vi "Buffer Statistics.vi"(0 "VISA resource name":refnum<visa-resource-name>, 5 "Channel (Channel A)":enum8{"Channel A", "Channel B"}(ring), 7 "Reading Buffer":string, 11 "error in (no error)":errorcluster) -> (4 "VISA resource name out":refnum<visa-resource-name>, 6 "Minimum Reading Details":string[](array[string]), 8 "Maximum Reading Details":string[](array[string]), 15 "error out":errorcluster)   [LabVIEW 2018, in "Keithley 2600 Series.lvlib"]
doc: "This Vi will return a table with statistical data about the data inserted into the buffer. \n\n<b>Functions and Attributes used</b>\nsmux.buffer.recalculatestats\nsmux.buffer.getstats"
uses:
  Keithley 2600 Series.lvlib
  Private/GlobalVariables.vi
panel:
  out "Statistics Undefined":bool
  out "Standard Deviation":dbl
  out "Mean":dbl
  out "Number of Data Points":u32
  # "(c) 2010 Keithley Instruments, Inc.  ALL RIGHTS RESERVED."
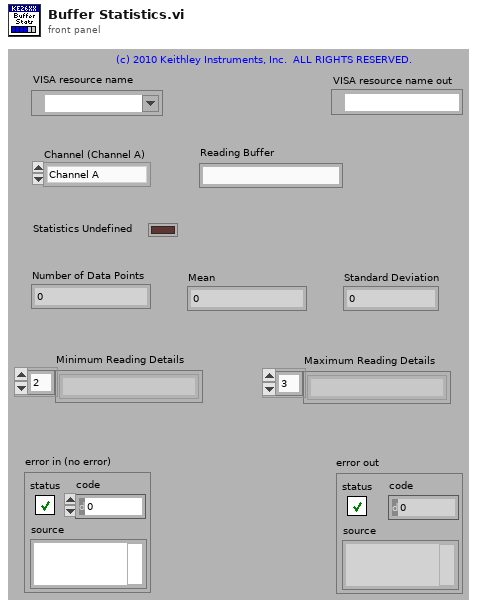
[diagram p1: front panel]
types:
  T1 = cluster{"[0]":dbl, "[1]":dbl, "[2]":dbl, "[3]":dbl, "[4]":dbl, "[5]":dbl, "[6]":dbl, "[7]":dbl, "[8]":dbl}
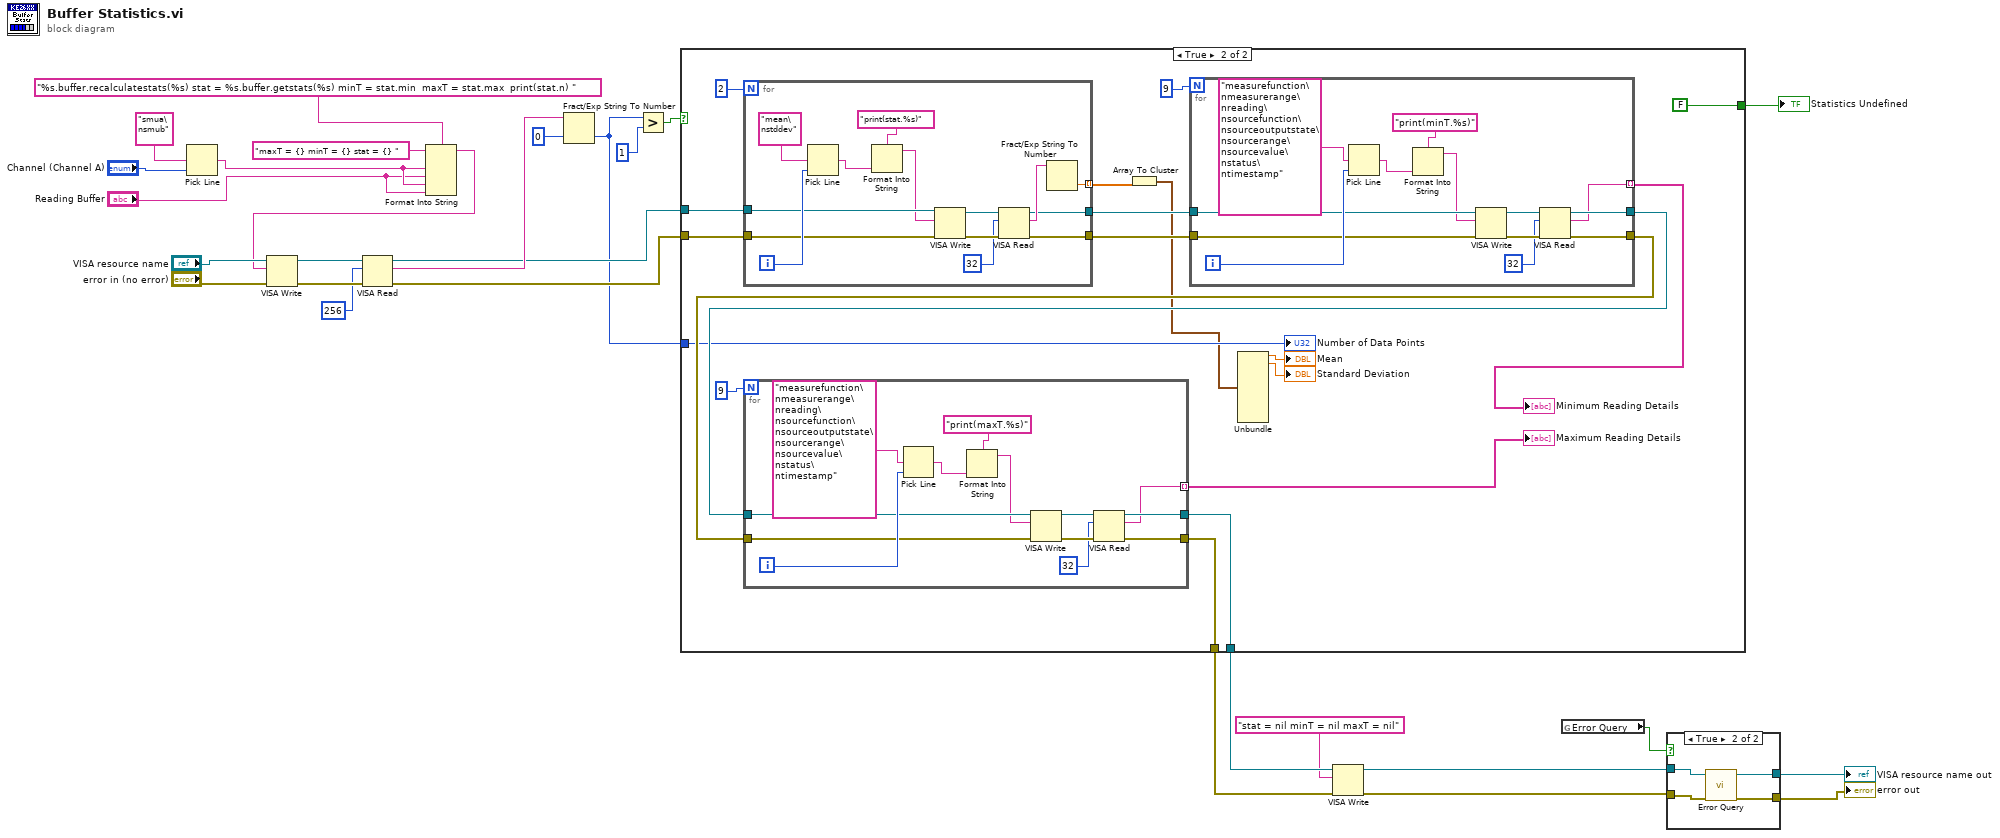
[diagram p0: block diagram]
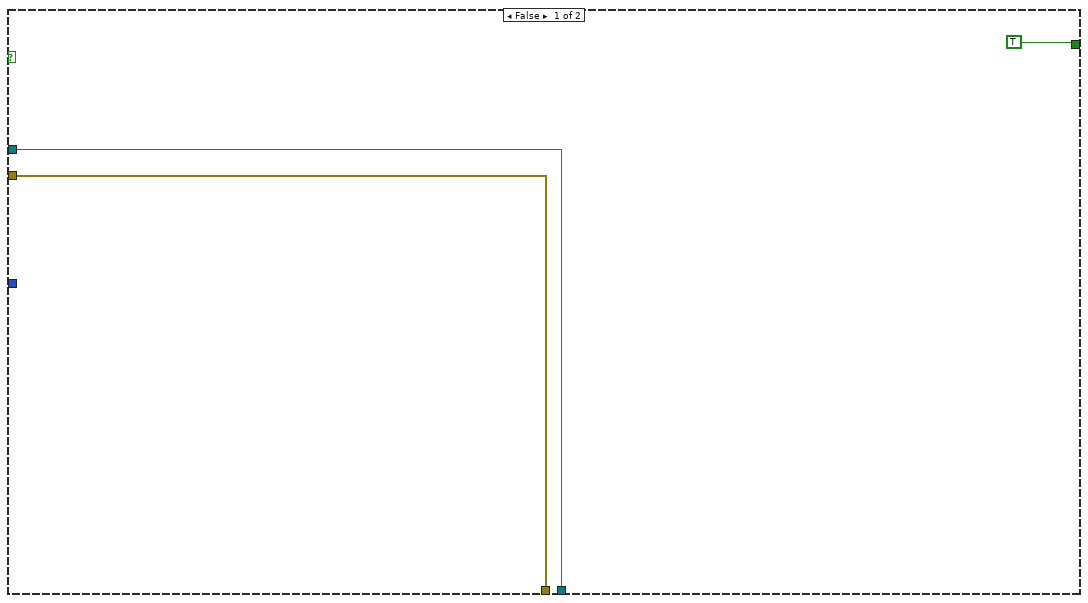
[diagram p2: hidden frame]
diagram:
  n1 = Pick Line(multi-line string="smua\nsmub", line index="Channel (Channel A)") -> (output string=w15:string)  [unwired: 1 in]
  n2 = Format Into String(format string="%s.buffer.recalculatestats(%s) stat = %s.buffer.getstats(%s) minT = stat.min  maxT = stat.max  print(stat.n) ", initial string="maxT = {} minT = {} stat = {} ", w15, "Reading Buffer", w15, "Reading Buffer") -> (resulting string=w16:string)  [unwired: 1 in, 1 out]
  n3 = VISA Write(VISA resource name="VISA resource name", write buffer=w16, error in (no error)="error in (no error)") -> (VISA resource name out=w24:refnum<visa-resource-name>, error out=w25:errorcluster)  [unwired: 1 out]
  n4 = VISA Read(VISA resource name=w24, byte count=u32 256, error in (no error)=w25) -> (VISA resource name out=w9:refnum<visa-resource-name>, read buffer=w13:string, error out=w8:errorcluster)  [unwired: 1 out]
  n5 = Fract/Exp String To Number(string=w13, default (0 dbl)=0) -> (number=w6:i32)  [unwired: 2 in, 1 out]
  n6 = Greater?(x=w6, y=1) -> (0:w10:bool)
  n7 = case shown="True" w10 {
    tunnel: w9 -> [w30 w50]
    tunnel: w8 -> [w29 w49]
    tunnel: w6 -> [_ w43]
    tunnel: [TRUE FALSE] -> w7
    tunnel: [w30 w38] -> w5
    tunnel: [w29 w37] -> w4
    frame False {
    }
    frame True {
      n8 = for {
        N: 2 -> [_]
        tunnel: w50 -> [w82]
        tunnel: w49 -> [w81]
        tunnel: [w79] -> w48 mode=indexing
        tunnel: [w78] -> w47
        tunnel: [w77] -> w46
        i -> [w85]
        n9 = Pick Line(multi-line string="mean\nstddev" ("initial string"), line index=w85) -> (output string=w84:string)  [unwired: 1 in]
        n10 = Format Into String(format string="print(stat.%s)" ("initial string"), w84) -> (resulting string=w80:string)  [unwired: 2 in, 1 out]
        n11 = VISA Write(VISA resource name=w82, write buffer=w80, error in (no error)=w81) -> (VISA resource name out=w89:refnum<visa-resource-name>, error out=w88:errorcluster)  [unwired: 1 out]
        n12 = VISA Read(VISA resource name=w89, byte count=u32 32, error in (no error)=w88) -> (VISA resource name out=w78:refnum<visa-resource-name>, read buffer=w90:string, error out=w77:errorcluster)  [unwired: 1 out]
        n13 = Fract/Exp String To Number(string=w90) -> (number=w79:dbl)  [unwired: 3 in, 1 out]
      }
      n14 = Array To Cluster(array=w48) -> (cluster=w42:T1)
      n15 = for {
        N: 9 -> [_]
        tunnel: w47 -> [w70]
        tunnel: w46 -> [w69]
        tunnel: [w64] -> w33 mode=indexing
        tunnel: [w67] -> w44
        tunnel: [w66] -> w45
        i -> [w73]
        n16 = Pick Line(multi-line string="measurefunction\nmeasurerange\nreading\nsourcefunction\nsourceoutputstate\nsourcerange\nsourcevalue\nstatus\ntimestamp", line index=w73) -> (output string=w72:string)  [unwired: 1 in]
        n17 = Format Into String(format string="print(minT.%s)" ("initial string"), w72) -> (resulting string=w68:string)  [unwired: 2 in, 1 out]
        n18 = VISA Write(VISA resource name=w70, write buffer=w68, error in (no error)=w69) -> (VISA resource name out=w76:refnum<visa-resource-name>, error out=w75:errorcluster)  [unwired: 1 out]
        n19 = VISA Read(VISA resource name=w76, byte count=u32 32, error in (no error)=w75) -> (VISA resource name out=w66:refnum<visa-resource-name>, read buffer=w64:string, error out=w67:errorcluster)  [unwired: 1 out]
      }
      "Minimum Reading Details" <- w33
      n20 = for {
        N: 9 -> [_]
        tunnel: w45 -> [w57]
        tunnel: w44 -> [w56]
        tunnel: [w51] -> w32 mode=indexing
        tunnel: [w54] -> w37
        tunnel: [w53] -> w38
        i -> [w60]
        n21 = Pick Line(multi-line string="measurefunction\nmeasurerange\nreading\nsourcefunction\nsourceoutputstate\nsourcerange\nsourcevalue\nstatus\ntimestamp", line index=w60) -> (output string=w59:string)  [unwired: 1 in]
        n22 = Format Into String(format string="print(maxT.%s)" ("initial string"), w59) -> (resulting string=w55:string)  [unwired: 2 in, 1 out]
        n23 = VISA Write(VISA resource name=w57, write buffer=w55, error in (no error)=w56) -> (VISA resource name out=w63:refnum<visa-resource-name>, error out=w62:errorcluster)  [unwired: 1 out]
        n24 = VISA Read(VISA resource name=w63, byte count=u32 32, error in (no error)=w62) -> (VISA resource name out=w53:refnum<visa-resource-name>, read buffer=w51:string, error out=w54:errorcluster)  [unwired: 1 out]
      }
      "Maximum Reading Details" <- w32
      n25 = Unbundle(w42) -> ("[0]"=→"Mean":dbl, "[1]"=→"Standard Deviation":dbl)  [unwired: 7 out]
      "Number of Data Points" <- w43
    }
  }
  "Statistics Undefined" <- w7
  n26 = VISA Write(VISA resource name=w5, write buffer="stat = nil minT = nil maxT = nil", error in (no error)=w4) -> (VISA resource name out=w2:refnum<visa-resource-name>, error out=w3:errorcluster)  [unwired: 1 out]
  n27 = global read "GlobalVariables.vi" "Error Query"() -> (w28:bool)
  n28 = case shown="True" w28 {
    tunnel: w2 -> [w92 w96]
    tunnel: w3 -> [w91 w95]
    tunnel: [w92 w94] -> w27
    tunnel: [w91 w93] -> w26
    frame False {
    }
    frame True {
      n29 = call "Error Query.vi"("error in (no error)"=w95, "VISA resource name"=w96) -> ("error out"=w93:errorcluster, "VISA resource name out"=w94:refnum<visa-resource-name>)  [unwired: 8 out]
    }
  }
  "VISA resource name out" <- w27
  "error out" <- w26
